vi "Process.vi"(8 "error in":errorcluster, 11 "Plugin in":refnum<class "AutomotiveDataSimulator.lvclass">) -> (0 "error out":errorcluster, 3 "Plugin out":refnum<class "AutomotiveDataSimulator.lvclass">)   [LabVIEW 2020, in "AutomotiveDataSimulator.lvlib" / "AutomotiveDataSimulator.lvclass"]
uses:
  AutomotiveDataSimulator.lvclass
  C:/Program Files/National Instruments/LabVIEW 2020/vi.lib/FlexLogger/SDK/PluginSDK.lvlibp/PEFClasses/SDK/Plugin/Plugin.lvclass
  AutomotiveDataSimulator.lvclass/AutomotiveDataSimulator.ctl
  <vilib>/numeric/Random Number (Range) DBL.vi
  <vilib>/FlexLogger/SDK/PluginSDK.lvlibp/PEFClasses/SDK/Plugin/DataHelpers/Write 1D DBL (NChan 1Sample).vi
  <vilib>/FlexLogger/SDK/PluginSDK.lvlibp/PEFClasses/SDK/Plugin/Plugin.lvclass
  C:/Program Files/National Instruments/LabVIEW 2020/vi.lib/FlexLogger/SDK/PluginSDK.lvlibp/PEFClasses/SDK/Processing Element/Processing Element.lvclass
  C:/Users/dgrajale/Desktop/Flexlogger Project/Flexlogger Plugins/AutomotiveDataSimulator/AutomotiveDataSimulator.lvclass
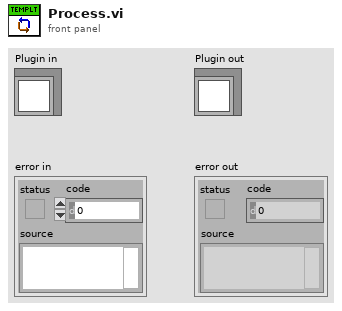
[diagram p1: front panel]
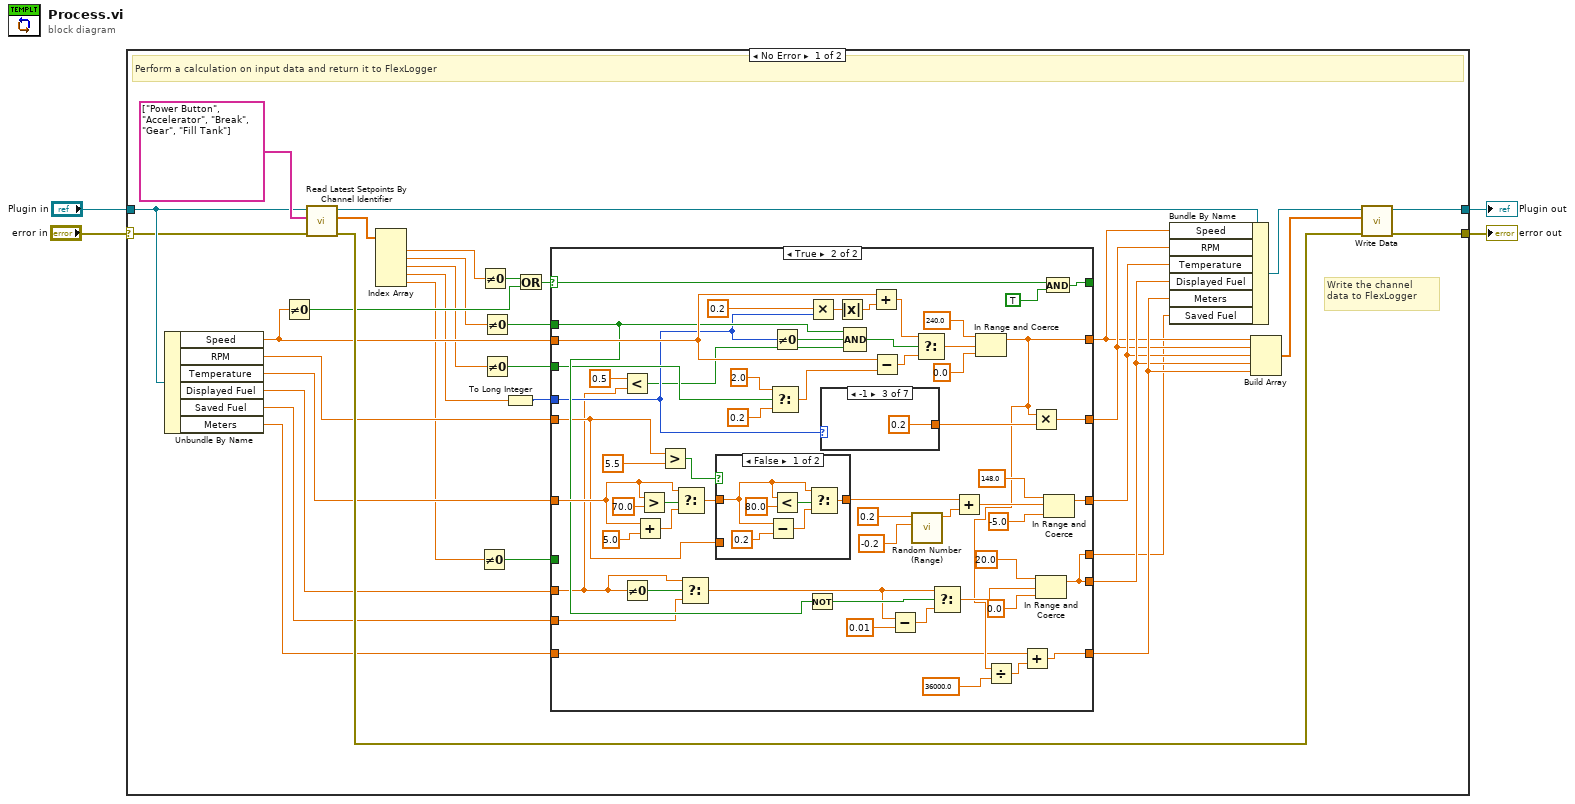
[diagram p0: block diagram]
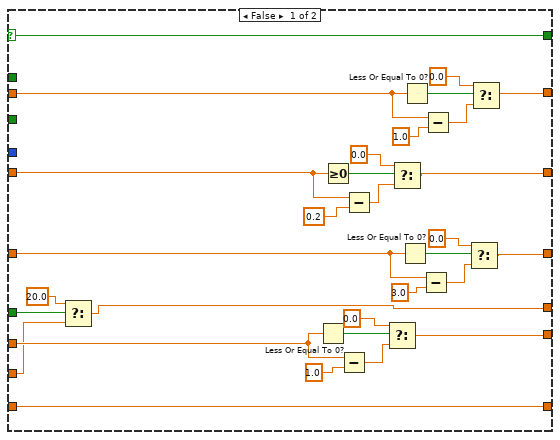
[diagram p2: hidden frame]
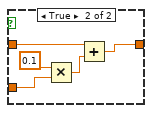
[diagram p3: hidden frame]
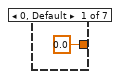
[diagram p4: hidden frame]
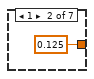
[diagram p5: hidden frame]
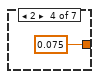
[diagram p6: hidden frame]
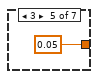
[diagram p7: hidden frame]
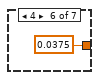
[diagram p8: hidden frame]
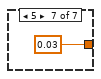
[diagram p9: hidden frame]
diagram:
  n1 = case shown="No Error" "error in" {
    selector: "error in" -> [w14 w144]
    tunnel: [w37 w145] -> w1
    tunnel: "Plugin in" -> [w15 w145]
    tunnel: [w38 w144] -> w2
    frame No Error {
      # "Write the channel data to FlexLogger"
      # "Perform a calculation on input data and return it to FlexLogger"
      n2 = Unbundle By Name(w15) -> ("Speed"=w32:dbl, "RPM"=w31:dbl, "Temperature"=w30:dbl, "Displayed Fuel"=w29:dbl, "Saved Fuel"=w17:dbl, "Meters"=w18:dbl)
      n3 = Not Equal To 0?(x=w32) -> (x != 0?=w34:bool)
      n4 = call <vilib>:"Read Latest Setpoints By Channel Identifier.vi"("error in (no error)"=w14, "Unique Channel Identifers (empty = all)"=string[] ["Power Button", "Accelerator", "Break", "Gear", "Fill Tank"], "Plugin in"=w15) -> ("error out"=w36:errorcluster, "Channel Setpoints"=w35:dbl[], "Plugin out"=w27:refnum<class "AutomotiveDataSimulator.lvclass">)  [unwired: 5 in, 1 out]
      n5 = Index Array(array=w35) -> (element #1=w9:dbl, element #2=w8:dbl, element #3=w7:dbl, element #4=w6:dbl, element #5=w5:dbl)  [unwired: 5 in]
      n6 = Not Equal To 0?(x=w5) -> (x != 0?=w10:bool)
      n7 = Not Equal To 0?(x=w9) -> (x != 0?=w13:bool)
      n8 = Not Equal To 0?(x=w8) -> (x != 0?=w12:bool)
      n9 = Not Equal To 0?(x=w7) -> (x != 0?=w11:bool)
      n10 = To Long Integer(number=w6) -> (32bit integer=w20:i32)
      n11 = Or(x=w13, y=w34) -> (x .or. y?=w33:bool)
      n12 = case shown="True" w33 {
        selector: w33 -> [w48 w112]
        tunnel: [w49 w78] -> w21
        tunnel: [w59 w98] -> w23
        tunnel: [w67 w83] -> w24
        tunnel: [w54 w114] -> w22
        tunnel: w32 -> [w50 w122]
        tunnel: w30 -> [w60 w103]
        tunnel: w29 -> [w66 w70]
        tunnel: w31 -> [w55 w71]
        tunnel: [w48 w111] -> _
        tunnel: w18 -> [w43 w77]
        tunnel: [w43 w76] -> w25
        tunnel: w10 -> [w42 _]
        tunnel: w12 -> [_ w87]
        tunnel: w20 -> [_ w73]
        tunnel: [w40 w83] -> w19
        tunnel: w17 -> [w39 w75]
        tunnel: w11 -> [_ w74]
        frame False {
          n13 = Select(t=20.0, s=w42, f=w39) -> (s? t:f=w40:dbl)
          n14 = Less Or Equal To 0?(x=w66) -> (x <= 0?=w68:bool)
          n15 = Greater Or Equal To 0?(x=w55) -> (x >= 0?=w58:bool)
          n16 = Subtract(x=w66, y=1.0) -> (x-y=w65:dbl)
          n17 = Subtract(x=w55, y=0.2) -> (x-y=w57:dbl)
          n18 = Select(t=0.0, s=w68, f=w65) -> (s? t:f=w67:dbl)
          n19 = Select(t=0.0, s=w58, f=w57) -> (s? t:f=w54:dbl)
          n20 = Less Or Equal To 0?(x=w60) -> (x <= 0?=w63:bool)
          n21 = Less Or Equal To 0?(x=w50) -> (x <= 0?=w53:bool)
          n22 = Subtract(x=w60, y=3.0) -> (x-y=w62:dbl)
          n23 = Subtract(x=w50, y=1.0) -> (x-y=w52:dbl)
          n24 = Select(t=0.0, s=w63, f=w62) -> (s? t:f=w59:dbl)
          n25 = Select(t=0.0, s=w53, f=w52) -> (s? t:f=w49:dbl)
        }
        frame True {
          n26 = Less?(x=0.5, y=w70) -> (x < y?=w69:bool)
          n27 = Not Equal To 0?(x=w70) -> (x != 0?=w82:bool)
          n28 = Add(x=w103, y=5.0) -> (x+y=w102:dbl)
          n29 = Greater?(x=w103, y=70.0 ("f")) -> (0:w106:bool)
          n30 = Greater?(x=w71, y=5.5) -> (0:w109:bool)
          n31 = Select(t=w103, s=w106, f=w102) -> (s? t:f=w105:dbl)
          n32 = Select(t=w70, s=w82, f=w75) -> (s? t:f=w81:dbl)
          n33 = case shown="False" w109 {
            tunnel: w105 -> [w127 w136]
            tunnel: [w126 w135] -> w107
            tunnel: w71 -> [_ w132]
            frame False {
              n34 = Subtract(x=w127, y=0.2) -> (x-y=w131:dbl)
              n35 = Less?(x=w127, y=80.0 ("f")) -> (x < y?=w130:bool)
              n36 = Select(t=w127, s=w130, f=w131) -> (s? t:f=w126:dbl)
            }
            frame True {
              n37 = Multiply(x=0.1 ("y"), y=w132) -> (x*y=w134:dbl)
              n38 = Add(x=w136, y=w134) -> (x+y=w135:dbl)
            }
          }
          n39 = Select(t=2.0, s=w74, f=0.2) -> (s? t:f=w118:dbl)
          n40 = Not Equal To 0?(x=w73) -> (x != 0?=w116:bool)
          n41 = Not(x=w87) -> (.not. x?=w88:bool)
          n42 = Multiply(x=0.2 ("y"), y=w73) -> (x*y=w85:dbl)
          n43 = case shown="-1" w73 {
            tunnel: [0.0 0.125 0.2 0.075 0.05 0.0375 0.03] -> w113
            frame 0, Default {
            }
            frame 1 {
            }
            frame -1 {
            }
            frame 2 {
            }
            frame 3 {
            }
            frame 4 {
            }
            frame 5 {
            }
          }
          n44 = Absolute Value(x=w85) -> (abs(x)=w84:dbl)
          n45 = Compound Arithmetic op=AND(w87, w116, w69) -> (w117:bool)
          n46 = Add(x=w122, y=w84) -> (x+y=w123:dbl)
          n47 = Subtract(x=w122, y=w118) -> (x-y=w121:dbl)
          n48 = Subtract(x=w81, y=0.01) -> (x-y=w90:dbl)
          n49 = call-poly <vilib>:"Random Number (Range).vi"("lower bound (0)"=-0.2, "upper bound (100)"=0.2) -> ("number"=w96:dbl)  [unwired: 9 in]
          n50 = Select(t=w123, s=w117, f=w121) -> (s? t:f=w115:dbl)
          n51 = Select(t=w81, s=w88, f=w90) -> (s? t:f=w89:dbl)
          n52 = Add(x=w107, y=w96) -> (x+y=w97:dbl)
          n53 = In Range and Coerce(upper limit=240.0, x=w115, lower limit=0.0) -> (coerced(x)=w78:dbl)  [unwired: 1 out]
          n54 = Divide(x=w78, y=36000.0 ("x")) -> (x/y=w79:dbl)
          n55 = Add(x=w77, y=w79) -> (x+y=w76:dbl)
          n56 = Multiply(x=w78, y=w113) -> (x*y=w114:dbl)
          n57 = In Range and Coerce(upper limit=20.0, x=w89, lower limit=0.0) -> (coerced(x)=w83:dbl)  [unwired: 1 out]
          n58 = And(x=w112, y=TRUE) -> (x .and. y?=w111:bool)
          n59 = In Range and Coerce(upper limit=148.0, x=w97, lower limit=-5.0) -> (coerced(x)=w98:dbl)  [unwired: 1 out]
        }
      }
      n60 = Bundle By Name(cluster=w27, "Speed"=w21, "RPM"=w22, "Temperature"=w23, "Displayed Fuel"=w24, "Meters"=w25, "Saved Fuel"=w19) -> (w26:refnum<class "AutomotiveDataSimulator.lvclass">)
      n61 = Build Array(w21, w22, w23, w24, w25) -> (w28:dbl[])
      n62 = call-poly <vilib>:"Write Data.vi"("error in (no error)"=w36, "Data"=w28, "Plugin in"=w26) -> ("error out"=w38:errorcluster, "Plugin out"=w37:refnum<class "AutomotiveDataSimulator.lvclass">)  [unwired: 7 in]
    }
    frame Error {
    }
  }
  "error out" <- w2
  "Plugin out" <- w1
